vi "Array Concatenation.vi"() -> ()   [LabVIEW 2019]
panel:
  out "Array 2":i32[](array[numeric])
  out "Numeric":i32
  out "Array":i32[](array[numeric])
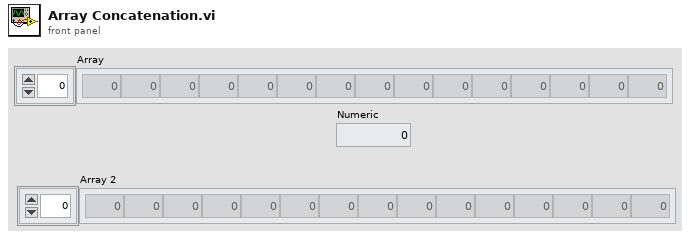
[diagram p1: front panel]
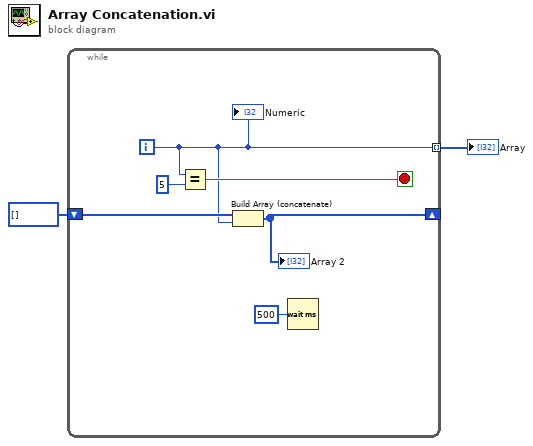
[diagram p0: block diagram]
diagram:
  n1 = while {
    tunnel: [w3] -> w2 mode=indexing
    shift-right: [w5] -> _
    shift-left: i32[] [] -> [w4]
    i -> [w3]
    stop <- w7 stop-if-true
    n2 = Equal?(x=w3, y=5) -> (x = y?=w7:bool)
    n3 = Build Array (concatenate)(w4, w3) -> (w5:i32[])
    "Array 2" <- w5
    n4 = Wait (ms)(milliseconds to wait=u32 500) -> ()  [unwired: 1 out]
    "Numeric" <- w3
  }
  "Array" <- w2
